vi "Update Test Server.vi"() -> ()   [LabVIEW 2013, in "OPC UA tests.lvlib"]
doc: "Forces the server to update every line in given input."
uses:
  OPC UA tests.lvlib
  module/configuration/OPC UA Data Type.ctl
  <vilib>/OPCUA/server/Write Bool.vi
  <vilib>/OPCUA/server/Write SByte.vi
  <vilib>/OPCUA/server/Write Byte.vi
  <vilib>/OPCUA/server/Write Int16.vi
  <vilib>/OPCUA/server/Write UInt16.vi
  <vilib>/OPCUA/server/Write Int32.vi
  <vilib>/OPCUA/server/Write UInt32.vi
  <vilib>/OPCUA/server/Write Int64.vi
  <vilib>/OPCUA/server/Write UInt64.vi
  <vilib>/OPCUA/server/Write Float.vi
  <vilib>/OPCUA/server/Write Double.vi
  <vilib>/OPCUA/server/Write String.vi
  <vilib>/OPCUA/server/Write Date Time.vi
  <vilib>/OPCUA/server/Write Bool Array.vi
  <vilib>/OPCUA/server/Write SByte Array.vi
  <vilib>/OPCUA/server/Write Byte Array.vi
  <vilib>/OPCUA/server/Write Int16 Array.vi
  <vilib>/OPCUA/server/Write UInt16 Array.vi
  <vilib>/OPCUA/server/Write Int32 Array.vi
  <vilib>/OPCUA/server/Write UInt32 Array.vi
  <vilib>/OPCUA/server/Write Int64 Array.vi
  <vilib>/OPCUA/server/Write UInt64 Array.vi
  <vilib>/OPCUA/server/Write Float Array.vi
  <vilib>/OPCUA/server/Write Double Array.vi
  <vilib>/OPCUA/server/Write String Array.vi
  <vilib>/OPCUA/server/Write Date Time Array.vi
  <vilib>/opcua/NI OPC UA Server.lvlib
  module/configuration/OPC UA configuration.lvclass
panel:
  out "error out":errorcluster
  in  "error in (no error)":errorcluster
  in  "OPC UA server refnum in":refnum<k21>
  in  "Items":cluster{"name":string, "OPC UA Data Type":T1}[](array[cluster]) {"OPC UA Data Type" items=["Boolean"=1, "SByte"=2, "Byte"=3, "Int16"=4, "UInt16"=5, "Int32"=6, "UInt32"=7, "Int64"=8, "UInt64"=9, "Float"=10, "Double"=11, "String"=12, "DateTime"=13, "ByteString"=15, "Array of Boolean"=101, "Array of SByte"=102, "Array of Byte"=103, "Array of Int16"=104, "Array of UInt16"=105, "Array of Int32"=106, "Array of UInt32"=107, "Array of Int64"=108, "Array of UInt64"=109, "Array of Float"=110, "Array of Double"=111, "Array of String"=112, "Array of DateTime"=113, "Array of ByteString"=115]}
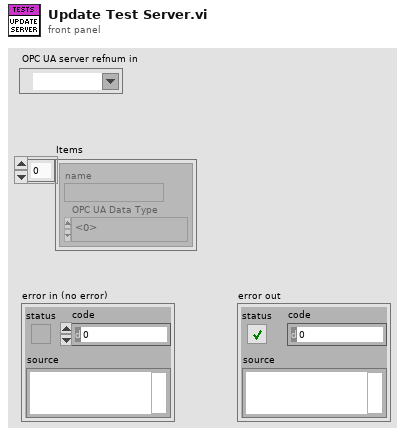
[diagram p1: front panel]
types:
  T1 = typedef "OPC UA configuration.lvclass/OPC UA Data Type.ctl" = u16
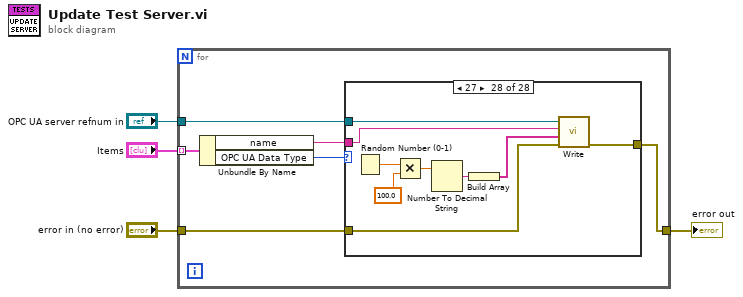
[diagram p0: block diagram]
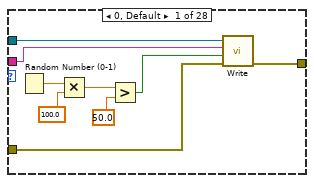
[diagram p2: hidden frame]
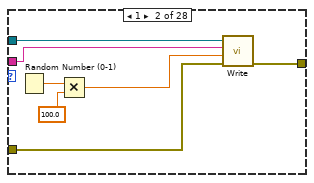
[diagram p3: hidden frame]
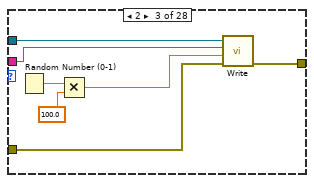
[diagram p4: hidden frame]
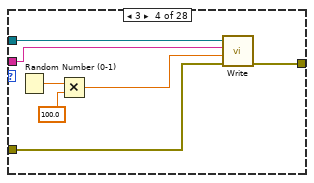
[diagram p5: hidden frame]
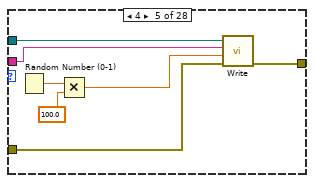
[diagram p6: hidden frame]
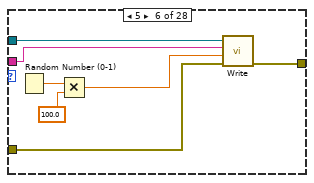
[diagram p7: hidden frame]
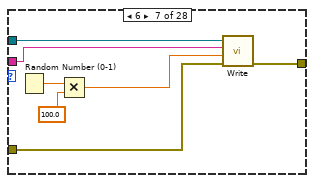
[diagram p8: hidden frame]
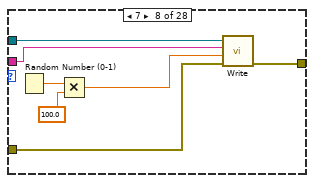
[diagram p9: hidden frame]
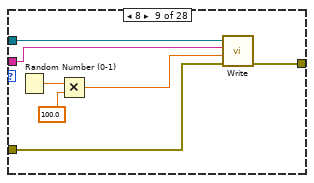
[diagram p10: hidden frame]
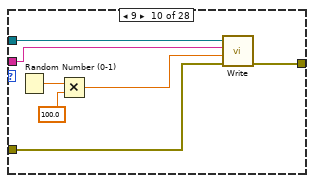
[diagram p11: hidden frame]
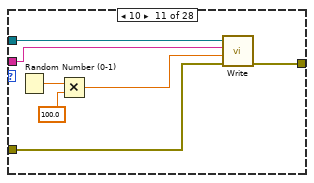
[diagram p12: hidden frame]
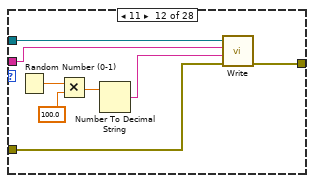
[diagram p13: hidden frame]
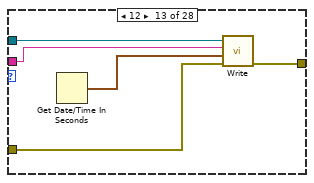
[diagram p14: hidden frame]
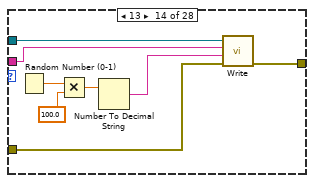
[diagram p15: hidden frame]
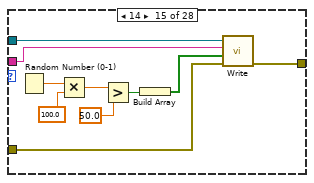
[diagram p16: hidden frame]
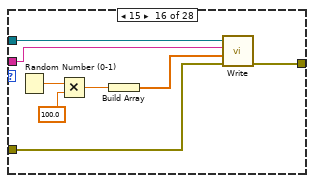
[diagram p17: hidden frame]
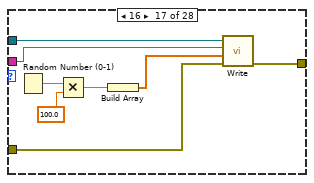
[diagram p18: hidden frame]
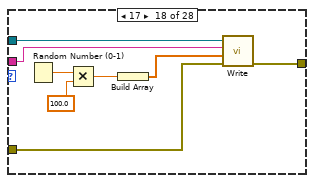
[diagram p19: hidden frame]
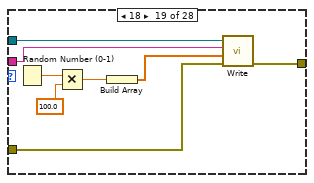
[diagram p20: hidden frame]
diagram:
  n1 = for {
    tunnel: "OPC UA server refnum in" -> [w10]
    tunnel: "Items" -> [w9] mode=indexing
    tunnel: "error in (no error)" -> [w6]
    tunnel: [w5] -> w1
    n2 = Unbundle By Name(w9) -> ("name"=w7:string, "OPC UA Data Type"=w8:T1)
    n3 = case shown="27" w8 {
      tunnel: w10 -> [w19 w26 w33 w40 w47 w54 w61 w68 w75 w82 w89 w97 w102 w110 w120 w128 w136 w144 w152 w160 w168 w176 w184 w192 w200 w209 w215 w224]
      tunnel: w7 -> [w18 w25 w32 w39 w46 w53 w60 w67 w74 w81 w88 w96 w101 w109 w119 w127 w135 w143 w151 w159 w167 w175 w183 w191 w199 w208 w214 w223]
      tunnel: w6 -> [w17 w24 w31 w38 w45 w52 w59 w66 w73 w80 w87 w95 w100 w108 w118 w126 w134 w142 w150 w158 w166 w174 w182 w190 w198 w207 w213 w222]
      tunnel: [w16 w23 w30 w37 w44 w51 w58 w65 w72 w79 w86 w94 w99 w107 w117 w125 w133 w141 w149 w157 w165 w173 w181 w189 w197 w206 w212 w221] -> w5
      frame 0, Default {
        n4 = Random Number (0-1)() -> (number: 0 to 1=w15:dbl)
        n5 = Multiply(x=w15, y=100.0) -> (x*y=w13:dbl)
        n6 = Greater?(x=w13, y=50.0) -> (0:w11:bool)
        n7 = call-poly <vilib>:"Write.vi"("error in (no error)"=w17, "value"=w11, "node path"=w18, "OPC UA server refnum in"=w19) -> ("error out"=w16:errorcluster)  [unwired: 6 in, 1 out]
      }
      frame 1 {
        n8 = Random Number (0-1)() -> (number: 0 to 1=w22:dbl)
        n9 = Multiply(x=w22, y=100.0) -> (x*y=w20:dbl)
        n10 = call-poly <vilib>:"Write.vi"("error in (no error)"=w24, "value"=w20, "node path"=w25, "OPC UA server refnum in"=w26) -> ("error out"=w23:errorcluster)  [unwired: 6 in, 1 out]
      }
      frame 2 {
        n11 = Random Number (0-1)() -> (number: 0 to 1=w29:dbl)
        n12 = Multiply(x=w29, y=100.0) -> (x*y=w27:dbl)
        n13 = call-poly <vilib>:"Write.vi"("error in (no error)"=w31, "value"=w27, "node path"=w32, "OPC UA server refnum in"=w33) -> ("error out"=w30:errorcluster)  [unwired: 6 in, 1 out]
      }
      frame 3 {
        n14 = Random Number (0-1)() -> (number: 0 to 1=w36:dbl)
        n15 = Multiply(x=w36, y=100.0) -> (x*y=w34:dbl)
        n16 = call-poly <vilib>:"Write.vi"("error in (no error)"=w38, "value"=w34, "node path"=w39, "OPC UA server refnum in"=w40) -> ("error out"=w37:errorcluster)  [unwired: 6 in, 1 out]
      }
      frame 4 {
        n17 = Random Number (0-1)() -> (number: 0 to 1=w43:dbl)
        n18 = Multiply(x=w43, y=100.0) -> (x*y=w41:dbl)
        n19 = call-poly <vilib>:"Write.vi"("error in (no error)"=w45, "value"=w41, "node path"=w46, "OPC UA server refnum in"=w47) -> ("error out"=w44:errorcluster)  [unwired: 6 in, 1 out]
      }
      frame 5 {
        n20 = Random Number (0-1)() -> (number: 0 to 1=w50:dbl)
        n21 = Multiply(x=w50, y=100.0) -> (x*y=w48:dbl)
        n22 = call-poly <vilib>:"Write.vi"("error in (no error)"=w52, "value"=w48, "node path"=w53, "OPC UA server refnum in"=w54) -> ("error out"=w51:errorcluster)  [unwired: 6 in, 1 out]
      }
      frame 6 {
        n23 = Random Number (0-1)() -> (number: 0 to 1=w57:dbl)
        n24 = Multiply(x=w57, y=100.0) -> (x*y=w55:dbl)
        n25 = call-poly <vilib>:"Write.vi"("error in (no error)"=w59, "value"=w55, "node path"=w60, "OPC UA server refnum in"=w61) -> ("error out"=w58:errorcluster)  [unwired: 6 in, 1 out]
      }
      frame 7 {
        n26 = Random Number (0-1)() -> (number: 0 to 1=w64:dbl)
        n27 = Multiply(x=w64, y=100.0) -> (x*y=w62:dbl)
        n28 = call-poly <vilib>:"Write.vi"("error in (no error)"=w66, "value"=w62, "node path"=w67, "OPC UA server refnum in"=w68) -> ("error out"=w65:errorcluster)  [unwired: 6 in, 1 out]
      }
      frame 8 {
        n29 = Random Number (0-1)() -> (number: 0 to 1=w71:dbl)
        n30 = Multiply(x=w71, y=100.0) -> (x*y=w69:dbl)
        n31 = call-poly <vilib>:"Write.vi"("error in (no error)"=w73, "value"=w69, "node path"=w74, "OPC UA server refnum in"=w75) -> ("error out"=w72:errorcluster)  [unwired: 6 in, 1 out]
      }
      frame 9 {
        n32 = Random Number (0-1)() -> (number: 0 to 1=w78:dbl)
        n33 = Multiply(x=w78, y=100.0) -> (x*y=w76:dbl)
        n34 = call-poly <vilib>:"Write.vi"("error in (no error)"=w80, "value"=w76, "node path"=w81, "OPC UA server refnum in"=w82) -> ("error out"=w79:errorcluster)  [unwired: 6 in, 1 out]
      }
      frame 10 {
        n35 = Random Number (0-1)() -> (number: 0 to 1=w85:dbl)
        n36 = Multiply(x=w85, y=100.0) -> (x*y=w83:dbl)
        n37 = call-poly <vilib>:"Write.vi"("error in (no error)"=w87, "value"=w83, "node path"=w88, "OPC UA server refnum in"=w89) -> ("error out"=w86:errorcluster)  [unwired: 6 in, 1 out]
      }
      frame 11 {
        n38 = Random Number (0-1)() -> (number: 0 to 1=w93:dbl)
        n39 = Multiply(x=w93, y=100.0) -> (x*y=w91:dbl)
        n40 = Number To Decimal String(number=w91) -> (decimal integer string=w90:string)  [unwired: 1 in]
        n41 = call-poly <vilib>:"Write.vi"("error in (no error)"=w95, "value"=w90, "node path"=w96, "OPC UA server refnum in"=w97) -> ("error out"=w94:errorcluster)  [unwired: 6 in, 1 out]
      }
      frame 12 {
        n42 = Get Date/Time In Seconds() -> (seconds since 1Jan1904=w98:timestamp)
        n43 = call-poly <vilib>:"Write.vi"("error in (no error)"=w100, "value"=w98, "node path"=w101, "OPC UA server refnum in"=w102) -> ("error out"=w99:errorcluster)  [unwired: 6 in, 1 out]
      }
      frame 13 {
        n44 = Random Number (0-1)() -> (number: 0 to 1=w106:dbl)
        n45 = Multiply(x=w106, y=100.0) -> (x*y=w104:dbl)
        n46 = Number To Decimal String(number=w104) -> (decimal integer string=w103:string)  [unwired: 1 in]
        n47 = call-poly <vilib>:"Write.vi"("error in (no error)"=w108, "value"=w103, "node path"=w109, "OPC UA server refnum in"=w110) -> ("error out"=w107:errorcluster)  [unwired: 6 in, 1 out]
      }
      frame 14 {
        n48 = Random Number (0-1)() -> (number: 0 to 1=w116:dbl)
        n49 = Multiply(x=w116, y=100.0) -> (x*y=w114:dbl)
        n50 = Greater?(x=w114, y=50.0) -> (0:w112:bool)
        n51 = Build Array(w112) -> (w111:bool[])
        n52 = call-poly <vilib>:"Write.vi"("error in (no error)"=w118, "value"=w111, "node path"=w119, "OPC UA server refnum in"=w120) -> ("error out"=w117:errorcluster)  [unwired: 6 in, 1 out]
      }
      frame 15 {
        n53 = Random Number (0-1)() -> (number: 0 to 1=w124:dbl)
        n54 = Multiply(x=w124, y=100.0) -> (x*y=w122:dbl)
        n55 = Build Array(w122) -> (w121:dbl[])
        n56 = call-poly <vilib>:"Write.vi"("error in (no error)"=w126, "value"=w121, "node path"=w127, "OPC UA server refnum in"=w128) -> ("error out"=w125:errorcluster)  [unwired: 6 in, 1 out]
      }
      frame 16 {
        n57 = Random Number (0-1)() -> (number: 0 to 1=w132:dbl)
        n58 = Multiply(x=w132, y=100.0) -> (x*y=w130:dbl)
        n59 = Build Array(w130) -> (w129:dbl[])
        n60 = call-poly <vilib>:"Write.vi"("error in (no error)"=w134, "value"=w129, "node path"=w135, "OPC UA server refnum in"=w136) -> ("error out"=w133:errorcluster)  [unwired: 6 in, 1 out]
      }
      frame 17 {
        n61 = Random Number (0-1)() -> (number: 0 to 1=w140:dbl)
        n62 = Multiply(x=w140, y=100.0) -> (x*y=w138:dbl)
        n63 = Build Array(w138) -> (w137:dbl[])
        n64 = call-poly <vilib>:"Write.vi"("error in (no error)"=w142, "value"=w137, "node path"=w143, "OPC UA server refnum in"=w144) -> ("error out"=w141:errorcluster)  [unwired: 6 in, 1 out]
      }
      frame 18 {
        n65 = Random Number (0-1)() -> (number: 0 to 1=w148:dbl)
        n66 = Multiply(x=w148, y=100.0) -> (x*y=w146:dbl)
        n67 = Build Array(w146) -> (w145:dbl[])
        n68 = call-poly <vilib>:"Write.vi"("error in (no error)"=w150, "value"=w145, "node path"=w151, "OPC UA server refnum in"=w152) -> ("error out"=w149:errorcluster)  [unwired: 6 in, 1 out]
      }
      frame 19 {
        n69 = Random Number (0-1)() -> (number: 0 to 1=w156:dbl)
        n70 = Multiply(x=w156, y=100.0) -> (x*y=w154:dbl)
        n71 = Build Array(w154) -> (w153:dbl[])
        n72 = call-poly <vilib>:"Write.vi"("error in (no error)"=w158, "value"=w153, "node path"=w159, "OPC UA server refnum in"=w160) -> ("error out"=w157:errorcluster)  [unwired: 6 in, 1 out]
      }
      frame 20 {
        n73 = Random Number (0-1)() -> (number: 0 to 1=w164:dbl)
        n74 = Multiply(x=w164, y=100.0) -> (x*y=w162:dbl)
        n75 = Build Array(w162) -> (w161:dbl[])
        n76 = call-poly <vilib>:"Write.vi"("error in (no error)"=w166, "value"=w161, "node path"=w167, "OPC UA server refnum in"=w168) -> ("error out"=w165:errorcluster)  [unwired: 6 in, 1 out]
      }
      frame 21 {
        n77 = Random Number (0-1)() -> (number: 0 to 1=w172:dbl)
        n78 = Multiply(x=w172, y=100.0) -> (x*y=w170:dbl)
        n79 = Build Array(w170) -> (w169:dbl[])
        n80 = call-poly <vilib>:"Write.vi"("error in (no error)"=w174, "value"=w169, "node path"=w175, "OPC UA server refnum in"=w176) -> ("error out"=w173:errorcluster)  [unwired: 6 in, 1 out]
      }
      frame 22 {
        n81 = Random Number (0-1)() -> (number: 0 to 1=w180:dbl)
        n82 = Multiply(x=w180, y=100.0) -> (x*y=w178:dbl)
        n83 = Build Array(w178) -> (w177:dbl[])
        n84 = call-poly <vilib>:"Write.vi"("error in (no error)"=w182, "value"=w177, "node path"=w183, "OPC UA server refnum in"=w184) -> ("error out"=w181:errorcluster)  [unwired: 6 in, 1 out]
      }
      frame 23 {
        n85 = Random Number (0-1)() -> (number: 0 to 1=w188:dbl)
        n86 = Multiply(x=w188, y=100.0) -> (x*y=w186:dbl)
        n87 = Build Array(w186) -> (w185:dbl[])
        n88 = call-poly <vilib>:"Write.vi"("error in (no error)"=w190, "value"=w185, "node path"=w191, "OPC UA server refnum in"=w192) -> ("error out"=w189:errorcluster)  [unwired: 6 in, 1 out]
      }
      frame 24 {
        n89 = Random Number (0-1)() -> (number: 0 to 1=w196:dbl)
        n90 = Multiply(x=w196, y=100.0) -> (x*y=w194:dbl)
        n91 = Build Array(w194) -> (w193:dbl[])
        n92 = call-poly <vilib>:"Write.vi"("error in (no error)"=w198, "value"=w193, "node path"=w199, "OPC UA server refnum in"=w200) -> ("error out"=w197:errorcluster)  [unwired: 6 in, 1 out]
      }
      frame 25 {
        n93 = Random Number (0-1)() -> (number: 0 to 1=w205:dbl)
        n94 = Multiply(x=w205, y=100.0) -> (x*y=w203:dbl)
        n95 = Number To Decimal String(number=w203) -> (decimal integer string=w202:string)  [unwired: 1 in]
        n96 = Build Array(w202) -> (w201:string[])
        n97 = call-poly <vilib>:"Write.vi"("error in (no error)"=w207, "value"=w201, "node path"=w208, "OPC UA server refnum in"=w209) -> ("error out"=w206:errorcluster)  [unwired: 6 in, 1 out]
      }
      frame 26 {
        n98 = Get Date/Time In Seconds() -> (seconds since 1Jan1904=w211:timestamp)
        n99 = Build Array(w211) -> (w210:timestamp[])
        n100 = call-poly <vilib>:"Write.vi"("error in (no error)"=w213, "value"=w210, "node path"=w214, "OPC UA server refnum in"=w215) -> ("error out"=w212:errorcluster)  [unwired: 6 in, 1 out]
      }
      frame 27 {
        n101 = Random Number (0-1)() -> (number: 0 to 1=w220:dbl)
        n102 = Multiply(x=w220, y=100.0) -> (x*y=w218:dbl)
        n103 = Number To Decimal String(number=w218) -> (decimal integer string=w217:string)  [unwired: 1 in]
        n104 = Build Array(w217) -> (w216:string[])
        n105 = call-poly <vilib>:"Write.vi"("error in (no error)"=w222, "value"=w216, "node path"=w223, "OPC UA server refnum in"=w224) -> ("error out"=w221:errorcluster)  [unwired: 6 in, 1 out]
      }
    }
  }
  "error out" <- w1
